vi "vars.vi"() -> ()   [LabVIEW 2020, in "Datron D4xxx.lvlib"]
uses:
  Datron D4xxx.lvlib
panel:
  in  "REN states VISAs":refnum<visa-resource-name>[](array[refnum])
  in  "REN states":u16[](array[ring]) items=["Local", "Remote"]
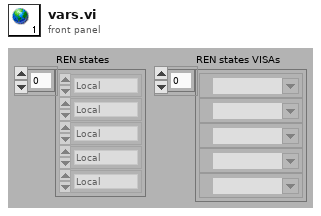
[diagram p1: front panel]
diagram:
